vi "Get_Indexes_and_Number_of_Jumps-3.vi"(4 "[IN] Minimal Subtrack\nLength for Making Desicion":i32, 5 "[IN] Index of connected\ntracks with problem dot":i32[](array[numeric]), 6 "[IN] Index of connected \ndots inside the track":i32[](array[numeric]), 7 "error IN":errorcluster, 8 "[IN] # of Track with\nFirst Problem Point":i32, 9 "[IN] Index of First Pro\nblem Point Inside Track":i32, 10 "[IN] Still connected\ntracks in group":T1) -> (0 "error OUT":errorcluster, 2 "[OUT] # of case":u8, 3 "[OUT] Indexes for Jumps":i32[](array[numeric]))   [LabVIEW 2013]
doc: "The subVI defines:\n- origin for \"11\" and \"111\" points; \n- saves 1st problem point; \n- searches the elongation of tracks and if it's problem point then saves its indicies \n(as 2nd and 3rd problem point)"
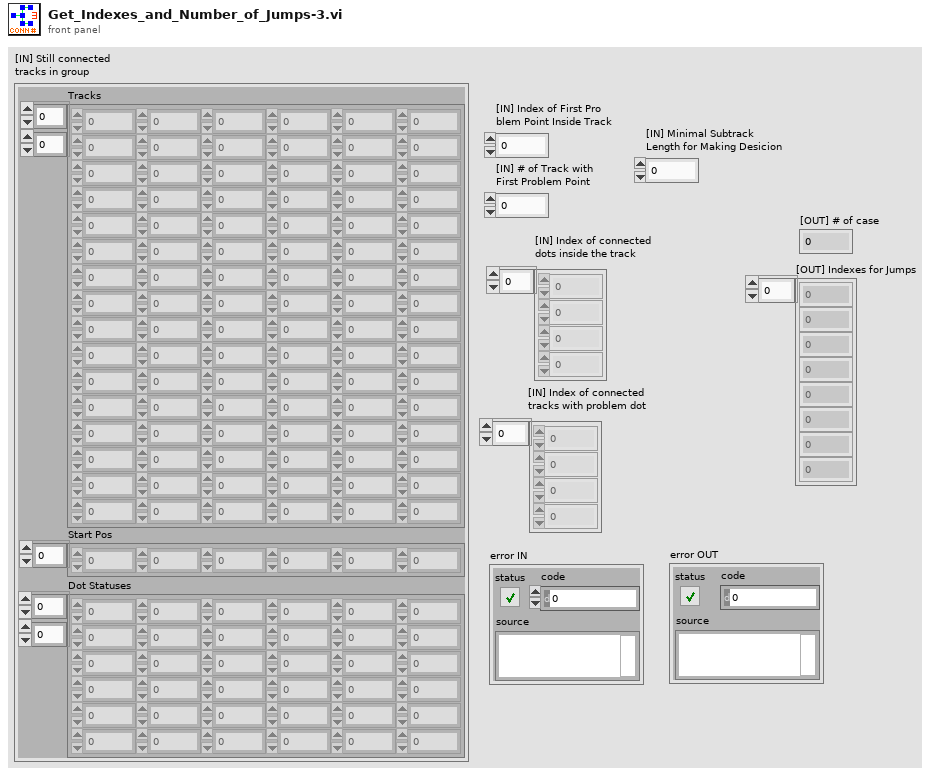
[diagram p1: front panel]
types:
  T1 = cluster{"Tracks":dbl[][], "Start Pos":i32[], "Dot Statuses":i16[][]}
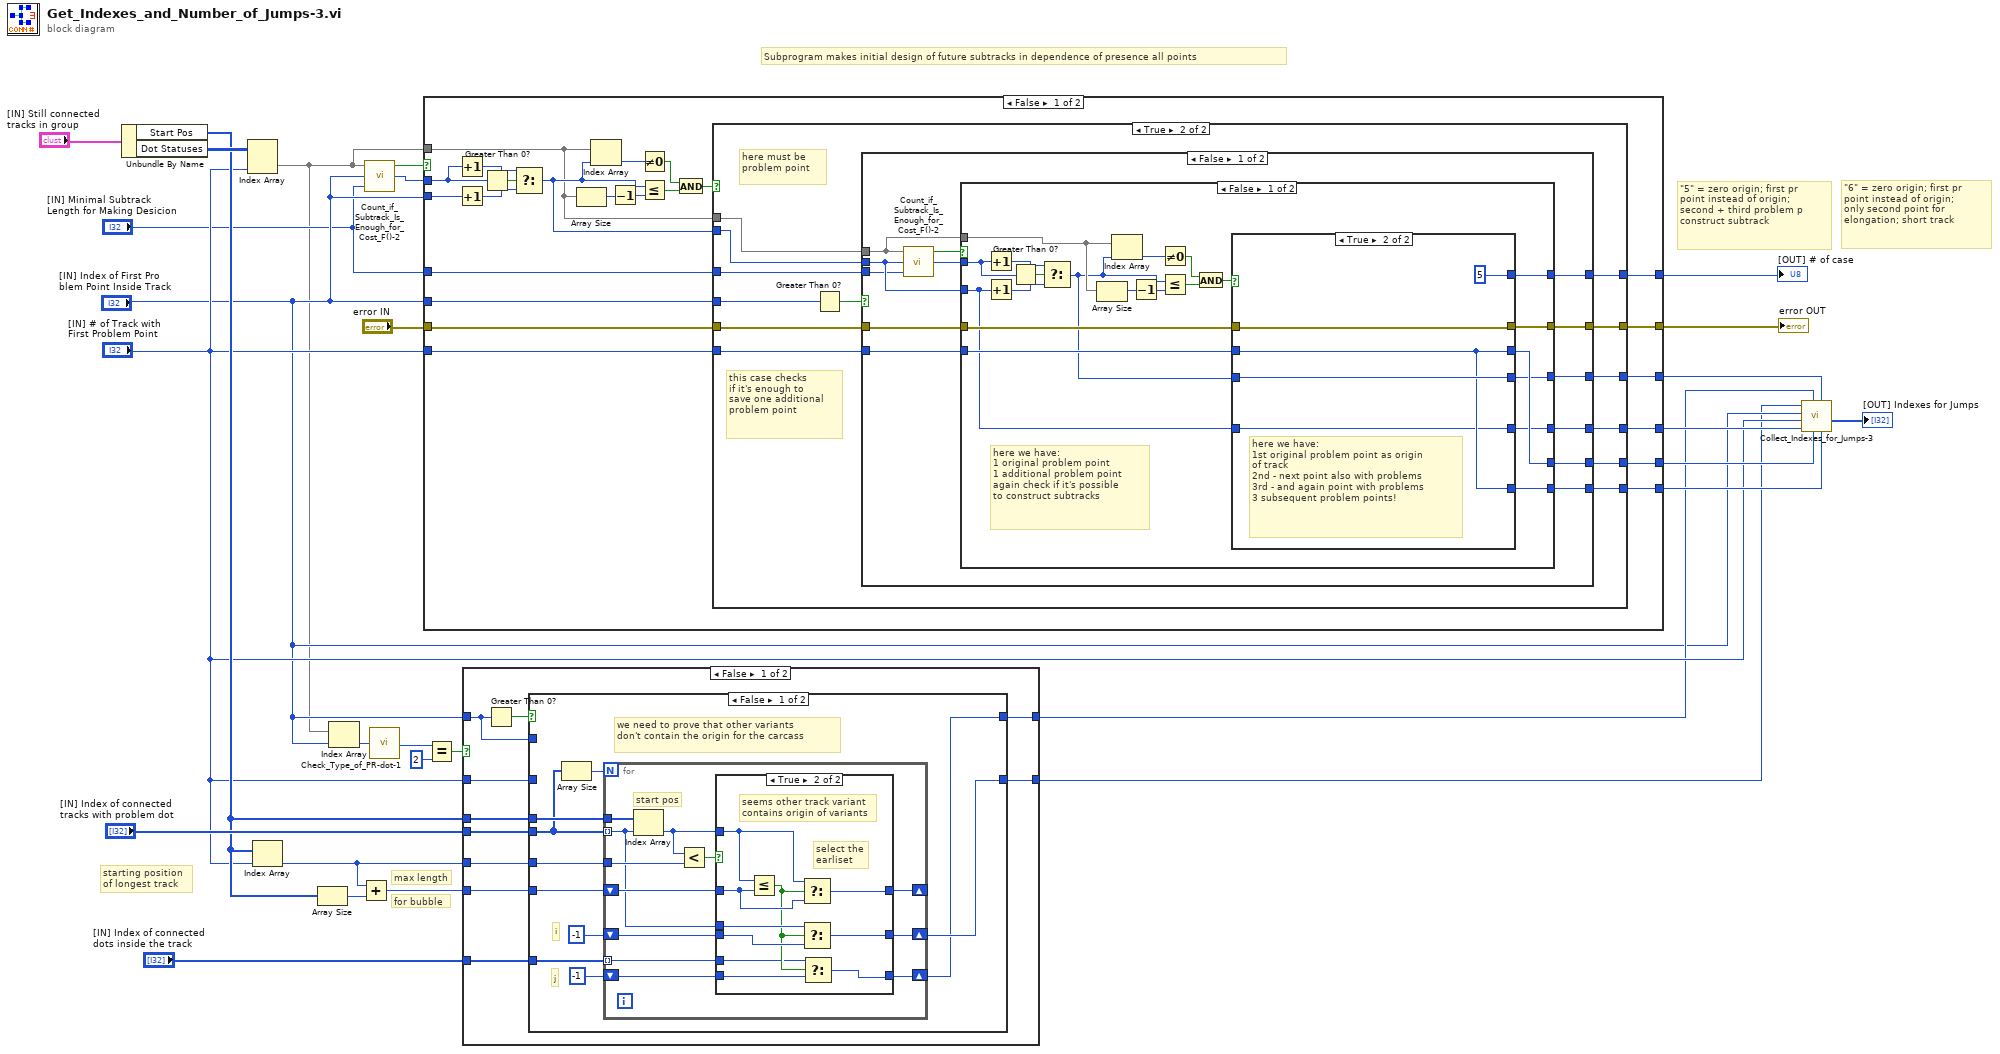
[diagram p0: block diagram]
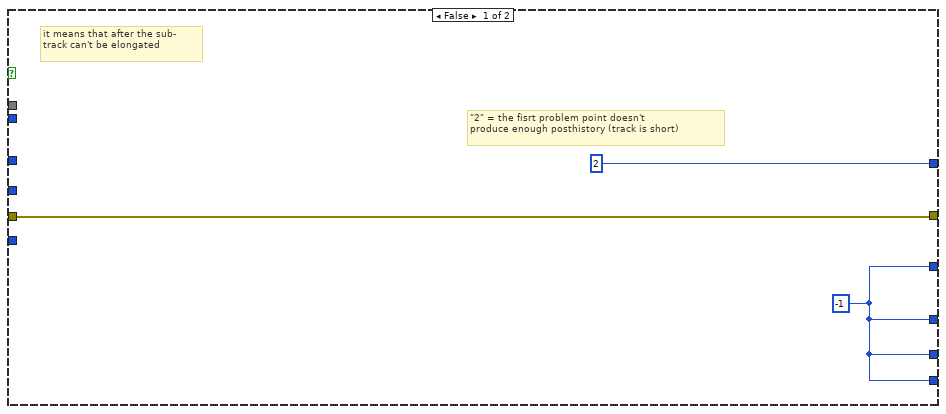
[diagram p5: hidden frame]
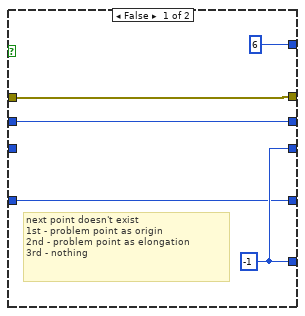
[diagram p6: hidden frame]
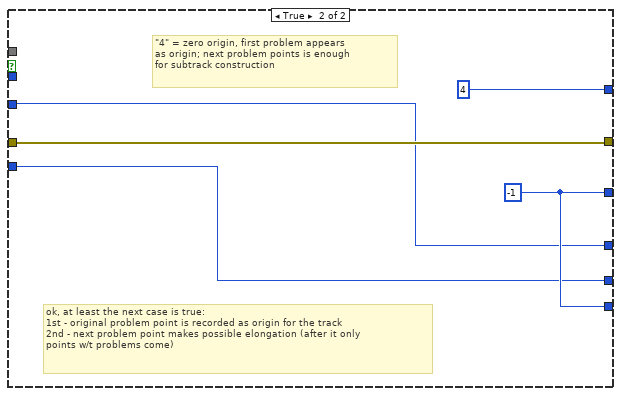
[diagram p7: hidden frame]
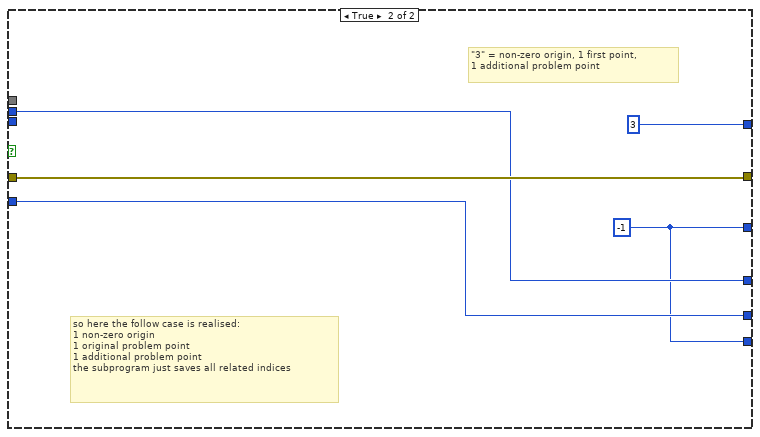
[diagram p8: hidden frame]
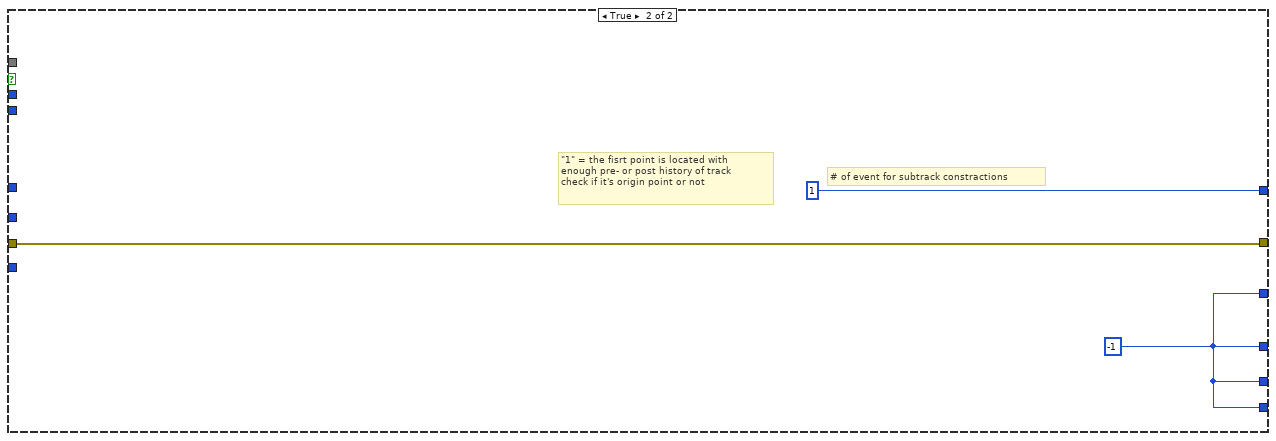
[diagram p9: hidden frame]
diagram:
  # "for bubble"
  # "max length"
  # "starting position \nof longest track"
  # "\"6\" = zero origin; first pr \npoint instead of origin; \nonly second point for \nelongation; short track"
  # "\"5\" = zero origin; first pr \npoint instead of origin; \nsecond + third problem p\nconstruct subtrack"
  # "Subprogram makes initial design of future subtracks in dependence of presence all points"
  n1 = Unbundle By Name("[IN] Still connected\ntracks in group") -> ("Start Pos"=w13:i32[], "Dot Statuses"=w27:i16[][])
  n2 = Index Array(array=w27, index (col)="[IN] # of Track with\nFirst Problem Point") -> (element=w4:i16[])  [unwired: 1 in]
  n3 = Index Array(array=w13, index="[IN] # of Track with\nFirst Problem Point") -> (element=w12:i32)
  n4 = Array Size(array=w13) -> (size(s)=w11:i32)
  n5 = Index Array(array=w4, index="[IN] Index of First Pro\nblem Point Inside Track") -> (element=w23:i16)
  n6 = Add(x=w12, y=w11) -> (x+y=w10:i32)
  n7 = call "Count_if_Subtrack_Is_Enough_for_Cost_F()-2.vi"("[IN] Minimal Subtrack Length \n(Points without problems) for\nMaking Desicion"="[IN] Minimal Subtrack\nLength for Making Desicion", "[IN] Index of Problem \nPoint Inside Track"="[IN] Index of First Pro\nblem Point Inside Track", "[IN] Dot Statuses in Track"=w4) -> ("[OUT] Index of Last \nPoint in Track"=w2:i32, "[OUT] It's enough to make\nconclusion using subtrack"=w3:bool)  [unwired: 1 in]
  n8 = call "Check_Type_of_PR-dot-1.vi"("[IN] dot status"=w23) -> ("[OUT] Type of\nproblem dot"=w22:i32)
  n9 = case shown="False" w3 {
    tunnel: w2 -> [w49 _]
    tunnel: "[IN] Index of First Pro\nblem Point Inside Track" -> [w47 _]
    tunnel: w4 -> [w37 _]
    tunnel: "[IN] Index of First Pro\nblem Point Inside Track" -> [w39 _]
    tunnel: "[IN] # of Track with\nFirst Problem Point" -> [w38 _]
    tunnel: "[IN] Minimal Subtrack\nLength for Making Desicion" -> [w36 _]
    tunnel: "error IN" -> [w35 w124]
    tunnel: [w34 w124] -> w25
    tunnel: [w33 u8 1] -> w24
    tunnel: [w31 w122] -> w19
    tunnel: [w30 w122] -> w18
    tunnel: [w32 w122] -> w17
    tunnel: [w29 w122] -> w16
    frame False {
      n10 = Increment(x=w49) -> (x+1=w50:i32)
      n11 = Increment(x=w47) -> (x+1=w48:i32)
      n12 = Greater Than 0?(x=w49) -> (x > 0?=w51:bool)
      n13 = Select(t=w50, s=w51, f=w48) -> (s? t:f=w40:i32)
      n14 = Array Size(array=w37) -> (size(s)=w46:i32)
      n15 = Index Array(array=w37, index=w40) -> (element=w43:i16)
      n16 = Decrement(x=w46) -> (x-1=w45:i32)
      n17 = Not Equal To 0?(x=w43) -> (x != 0?=w42:bool)
      n18 = Less Or Equal?(x=w40, y=w45) -> (x <= y?=w44:bool)
      n19 = And(x=w42, y=w44) -> (x .and. y?=w41:bool)
      n20 = case shown="True" w41 {
        tunnel: w40 -> [_ w64]
        tunnel: w39 -> [_ w63]
        tunnel: w38 -> [_ w67]
        tunnel: w37 -> [_ w66]
        tunnel: w36 -> [_ w65]
        tunnel: w35 -> [w54 w61]
        tunnel: [w54 w60] -> w34
        tunnel: [u8 2 w59] -> w33
        tunnel: [w52 w56] -> w32
        tunnel: [w52 w58] -> w31
        tunnel: [w52 w57] -> w30
        tunnel: [w52 w55] -> w29
        frame False {
          w52 = -1
          # "\"2\" = the fisrt problem point doesn't \nproduce enough posthistory (track is short)"
          # "it means that after the sub-\ntrack can't be elongated"
        }
        frame True {
          # "this case checks\nif it's enough to\nsave one additional\nproblem point"
          # "here must be \nproblem point"
          n21 = Greater Than 0?(x=w63) -> (x > 0?=w62:bool)
          n22 = case shown="False" w62 {
            tunnel: w67 -> [w78 w118]
            tunnel: w66 -> [w72 _]
            tunnel: w65 -> [w70 _]
            tunnel: w64 -> [w71 w119]
            tunnel: w61 -> [w80 w121]
            tunnel: [w79 w121] -> w60
            tunnel: [w77 u8 3] -> w59
            tunnel: [w74 w119] -> w58
            tunnel: [w73 w118] -> w57
            tunnel: [w76 w117] -> w56
            tunnel: [w75 w117] -> w55
            frame False {
              n23 = call "Count_if_Subtrack_Is_Enough_for_Cost_F()-2.vi"("[IN] Minimal Subtrack Length \n(Points without problems) for\nMaking Desicion"=w70, "[IN] Index of Problem \nPoint Inside Track"=w71, "[IN] Dot Statuses in Track"=w72) -> ("[OUT] Index of Last \nPoint in Track"=w69:i32, "[OUT] It's enough to make\nconclusion using subtrack"=w68:bool)  [unwired: 1 in]
              n24 = case shown="False" w68 {
                tunnel: w69 -> [w98 _]
                tunnel: w71 -> [w81 w112]
                tunnel: w72 -> [w92 _]
                tunnel: w80 -> [w90 w116]
                tunnel: [w89 w116] -> w79
                tunnel: w78 -> [w88 w113]
                tunnel: [w86 u8 4] -> w77
                tunnel: [w84 w114] -> w76
                tunnel: [w83 w114] -> w75
                tunnel: [w82 w112] -> w74
                tunnel: [w85 w113] -> w73
                frame False {
                  # "here we have:\n1 original problem point\n1 additional problem point\nagain check if it's possible \nto construct subtracks"
                  n25 = Increment(x=w98) -> (x+1=w100:i32)
                  n26 = Increment(x=w81) -> (x+1=w99:i32)
                  n27 = Greater Than 0?(x=w98) -> (x > 0?=w101:bool)
                  n28 = Select(t=w100, s=w101, f=w99) -> (s? t:f=w87:i32)
                  n29 = Array Size(array=w92) -> (size(s)=w97:i32)
                  n30 = Index Array(array=w92, index=w87) -> (element=w94:i16)
                  n31 = Decrement(x=w97) -> (x-1=w96:i32)
                  n32 = Not Equal To 0?(x=w94) -> (x != 0?=w93:bool)
                  n33 = Less Or Equal?(x=w87, y=w96) -> (x <= y?=w95:bool)
                  n34 = And(x=w93, y=w95) -> (x .and. y?=w91:bool)
                  n35 = case shown="True" w91 {
                    tunnel: [w106 w111] -> w89
                    tunnel: w90 -> [w106 w111]
                    tunnel: w88 -> [w104 w108]
                    tunnel: w87 -> [_ w109]
                    tunnel: [u8 6 u8 5] -> w86
                    tunnel: [w104 w108] -> w85
                    tunnel: [w103 w109] -> w84
                    tunnel: [w103 w108] -> w83
                    tunnel: [w102 w107] -> w82
                    tunnel: w81 -> [w102 w107]
                    frame False {
                      w103 = -1 ("[IN] # of Track with\nFirst Problem Point")
                      # "next point doesn't exist\n1st - problem point as origin\n2nd - problem point as elongation\n3rd - nothing"
                    }
                    frame True {
                      # "here we have:\n1st original problem point as origin\nof track\n2nd - next point also with problems\n3rd - and again point with problems\n3 subsequent problem points!"
                    }
                  }
                }
                frame True {
                  w114 = -1
                  # "\"4\" = zero origin, first problem appears\nas origin; next problem points is enough \nfor subtrack construction"
                  # "ok, at least the next case is true: \n1st - original problem point is recorded as origin for the track\n2nd - next problem point makes possible elongation (after it only \npoints w/t problems come)"
                }
              }
            }
            frame True {
              w117 = -1
              # "\"3\" = non-zero origin, 1 first point, \n1 additional problem point"
              # "so here the follow case is realised:\n1 non-zero origin \n1 original problem point\n1 additional problem point\nthe subprogram just saves all related indices"
            }
          }
        }
      }
    }
    frame True {
      w122 = -1
      # "\"1\" = the fisrt point is located with \nenough pre- or post history of track\ncheck if it's origin point or not"
      # "# of event for subtrack constractions"
    }
  }
  "error OUT" <- w25
  "[OUT] # of case" <- w24
  n36 = Equal?(x=w22, y=2) -> (x = y?=w20:bool)
  n37 = case shown="False" w20 {
    tunnel: [w132 w172] -> w8
    tunnel: "[IN] Index of First Pro\nblem Point Inside Track" -> [w133 w172]
    tunnel: [w130 w173] -> w1
    tunnel: "[IN] # of Track with\nFirst Problem Point" -> [w131 w173]
    tunnel: "[IN] Index of connected\ntracks with problem dot" -> [w129 _]
    tunnel: w12 -> [w128 _]
    tunnel: w13 -> [w127 _]
    tunnel: w10 -> [w126 _]
    tunnel: "[IN] Index of connected \ndots inside the track" -> [w125 _]
    frame False {
      n38 = Greater Than 0?(x=w133) -> (x > 0?=w134:bool)
      n39 = case shown="False" w134 {
        tunnel: w133 -> [_ w170]
        tunnel: [w135 w170] -> w132
        tunnel: w131 -> [_ w171]
        tunnel: [w138 w171] -> w130
        tunnel: w129 -> [w141 _]
        tunnel: w128 -> [w143 _]
        tunnel: w127 -> [w142 _]
        tunnel: w126 -> [w140 _]
        tunnel: w125 -> [w136 _]
        frame False {
          # "j"
          # "i"
          # "we need to prove that other variants\ndon't contain the origin for the carcass"
          n40 = Array Size(array=w141) -> (size(s)=w144:i32)
          n41 = for {
            N: w144 -> [_]
            tunnel: w141 -> [w148] mode=indexing
            tunnel: w143 -> [w155]
            tunnel: w142 -> [w156]
            shift-right: [w152] -> _
            shift-left: w140 -> [w153]
            shift-right: [w149] -> w138
            shift-left: -1 -> [w150]
            shift-right: [w145] -> w135
            shift-left: -1 -> [w147]
            tunnel: w136 -> [w146] mode=indexing
            # "start pos"
            n42 = Index Array(array=w156, index=w148) -> (element=w151:i32)
            n43 = Less?(x=w151, y=w155) -> (x < y?=w154:bool)
            n44 = case shown="True" w154 {
              tunnel: w153 -> [w159 w167]
              tunnel: [w159 w169] -> w152
              tunnel: w151 -> [_ w168]
              tunnel: w150 -> [w158 w165]
              tunnel: [w158 w164] -> w149
              tunnel: w148 -> [_ w166]
              tunnel: w147 -> [w157 w161]
              tunnel: w146 -> [_ w162]
              tunnel: [w157 w160] -> w145
              frame False {
              }
              frame True {
                # "select the \nearliset"
                # "seems other track variant\ncontains origin of variants"
                n45 = Less Or Equal?(x=w168, y=w167) -> (x <= y?=w163:bool)
                n46 = Select(t=w168, s=w163, f=w167) -> (s? t:f=w169:i32)
                n47 = Select(t=w166, s=w163, f=w165) -> (s? t:f=w164:i32)
                n48 = Select(t=w162, s=w163, f=w161) -> (s? t:f=w160:i32)
              }
            }
          }
        }
        frame True {
          # "so this subtrack already contains the origin"
        }
      }
    }
    frame True {
    }
  }
  n49 = call "Collect_Indexes_for_Jumps-3.vi"("[IN] # Track with \nThird Problem Point"=w16, "[IN] Index of Third\nProblem point"=w17, "[IN] # Track with \nSecond Problem Point"=w18, "[IN] Index of Point Be\nfore Problem (Origin)"=w8, "[IN] Index of Second\nProblem point"=w19, "[IN] # Track with First\nProblem Point"="[IN] # of Track with\nFirst Problem Point", "[IN] Index of First \nProblem Point"="[IN] Index of First Pro\nblem Point Inside Track", "[IN] # Track of Origin"=w1) -> ("[OUT] Indexes for Jumps"=→"[OUT] Indexes for Jumps":i32[])  [unwired: 3 in]
